vi "random shoot.vi"(10 "empty rounds":u32, 11 "live rounds":u32) -> (3 "Boolean":bool)   [LabVIEW 2025]
doc: "Decide who to shoot under unknown condition"
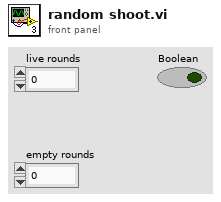
[diagram p1: front panel]
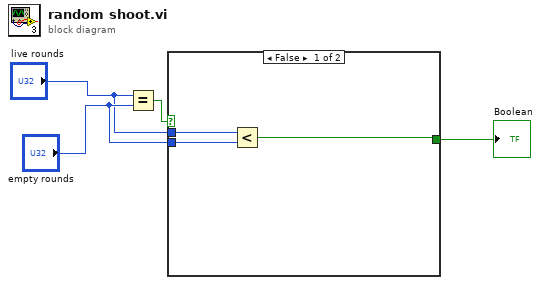
[diagram p0: block diagram]
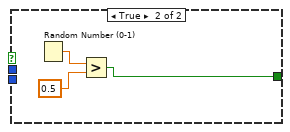
[diagram p2: hidden frame]
diagram:
  n1 = Equal?(x="live rounds", y="empty rounds") -> (x = y?=w1:bool)
  n2 = case shown="False" w1 {
    tunnel: [w5 w8] -> w2
    tunnel: "live rounds" -> [w7 _]
    tunnel: "empty rounds" -> [w6 _]
    frame False {
      n3 = Less?(x=w7, y=w6) -> (x < y?=w5:bool)
    }
    frame True {
      n4 = Random Number (0-1)() -> (number: 0 to 1=w10:dbl)
      n5 = Greater?(x=w10, y=0.5) -> (0:w8:bool)
    }
  }
  "Boolean" <- w2
